vi "TrendsD04.vi"() -> ()   [LabVIEW 2019, in "D04.lvlib"]
uses:
  D04.lvlib
  <vilib>/measure/mamon.llb/Trigger Detection for 1 Channel.vi
  <vilib>/measure/NI_MAPro.lvlib
panel:
  out "No Change":bool
  out "Sudden Change":bool
  out "Decrease":bool
  out "Increase":bool
  out "Previous  ES":dbl
  out "Present  Speed":dbl
  out "Present Error":dbl format="%#.2g"
  out "Previous Error":dbl
  out "Previous  Speed":dbl
  out "Previous PW":dbl caption="Control Information"
  out "Pulse Trends":waveform(i16)[](graph) caption="Waveform Chart - Dark"
  in  "Close":bool
  out "disc name":string="Disc 04 Trends"
  out "dsgs":string="DSGS"
  out "Speed Trend":waveform(dbl)(graph) caption="Waveform Chart - Dark"
  out "Average Trend":waveform(dbl)[](graph) caption="Waveform Chart - Dark"
  out "Live Trend":waveform(dbl)[](graph) caption="Waveform Chart - Dark"
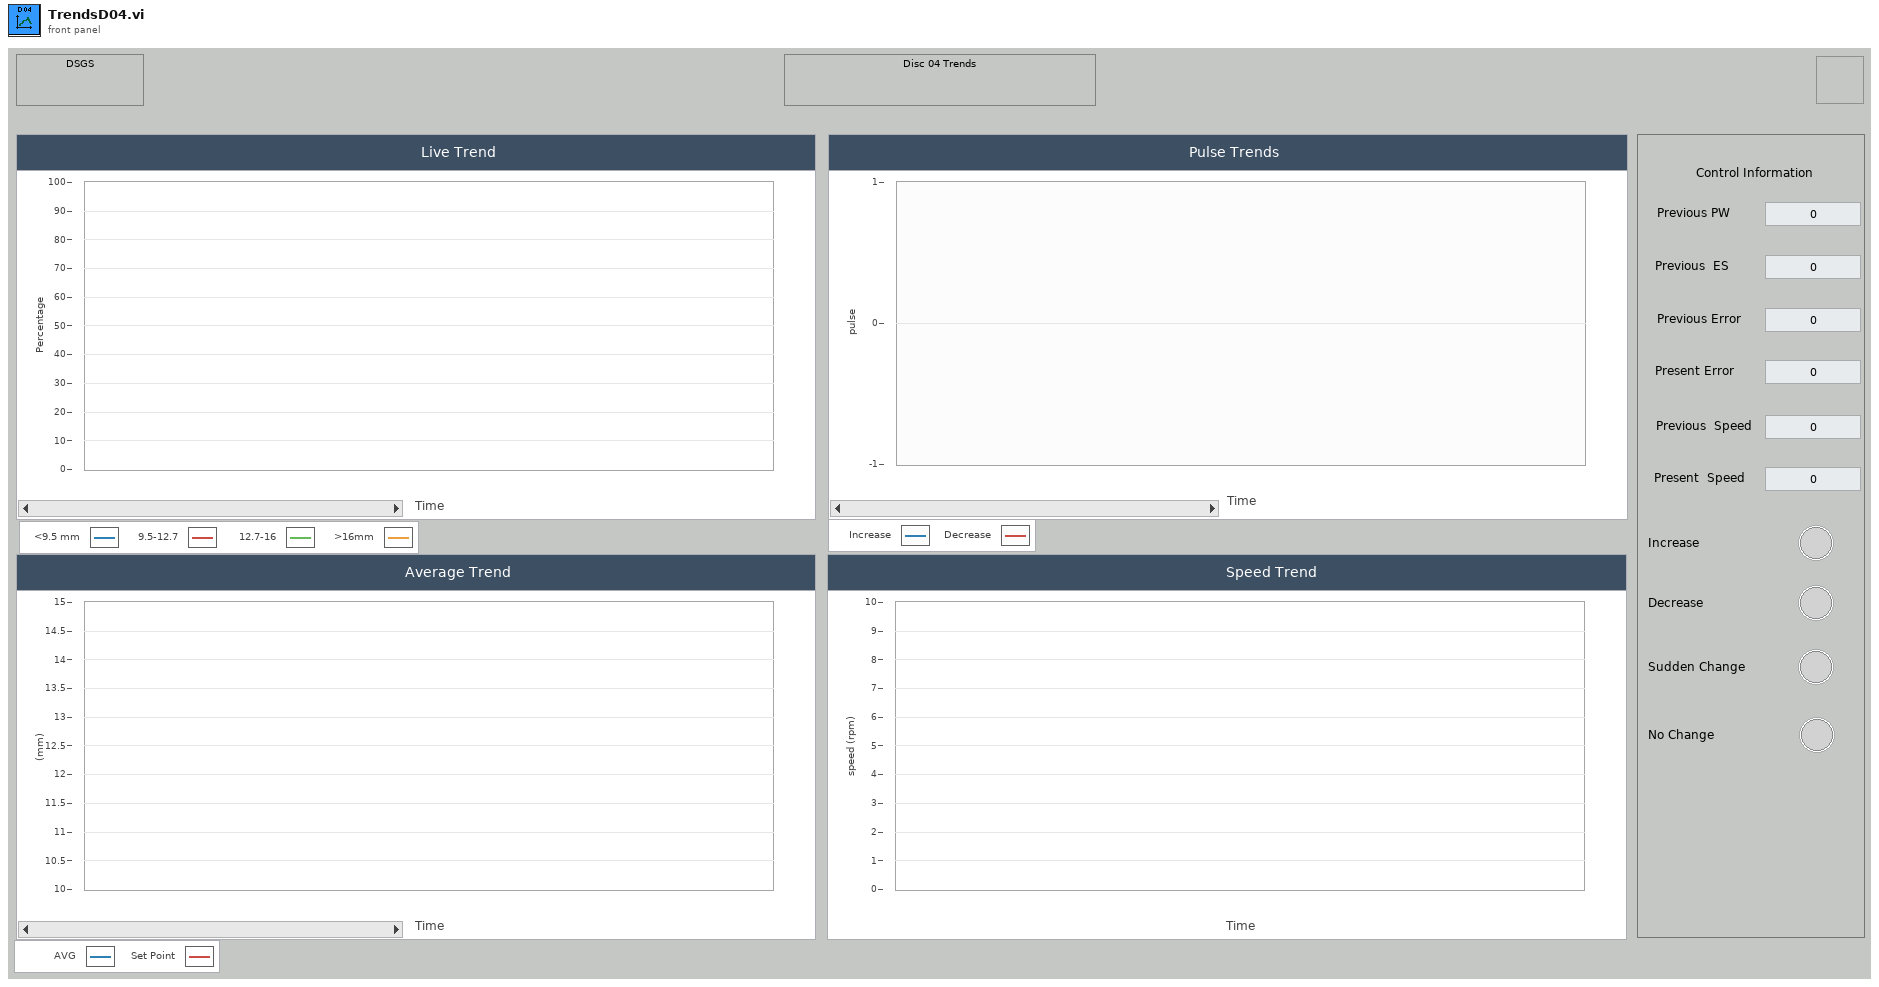
[diagram p1: front panel]
types:
  T1 = cluster{"decrease D04":bool, "increase D04":bool, "no change D04":bool, "sudden change D04":bool, "last error 04":dbl, "previouse speed D04":dbl, "pulse width D04":dbl, "slope D04":dbl}
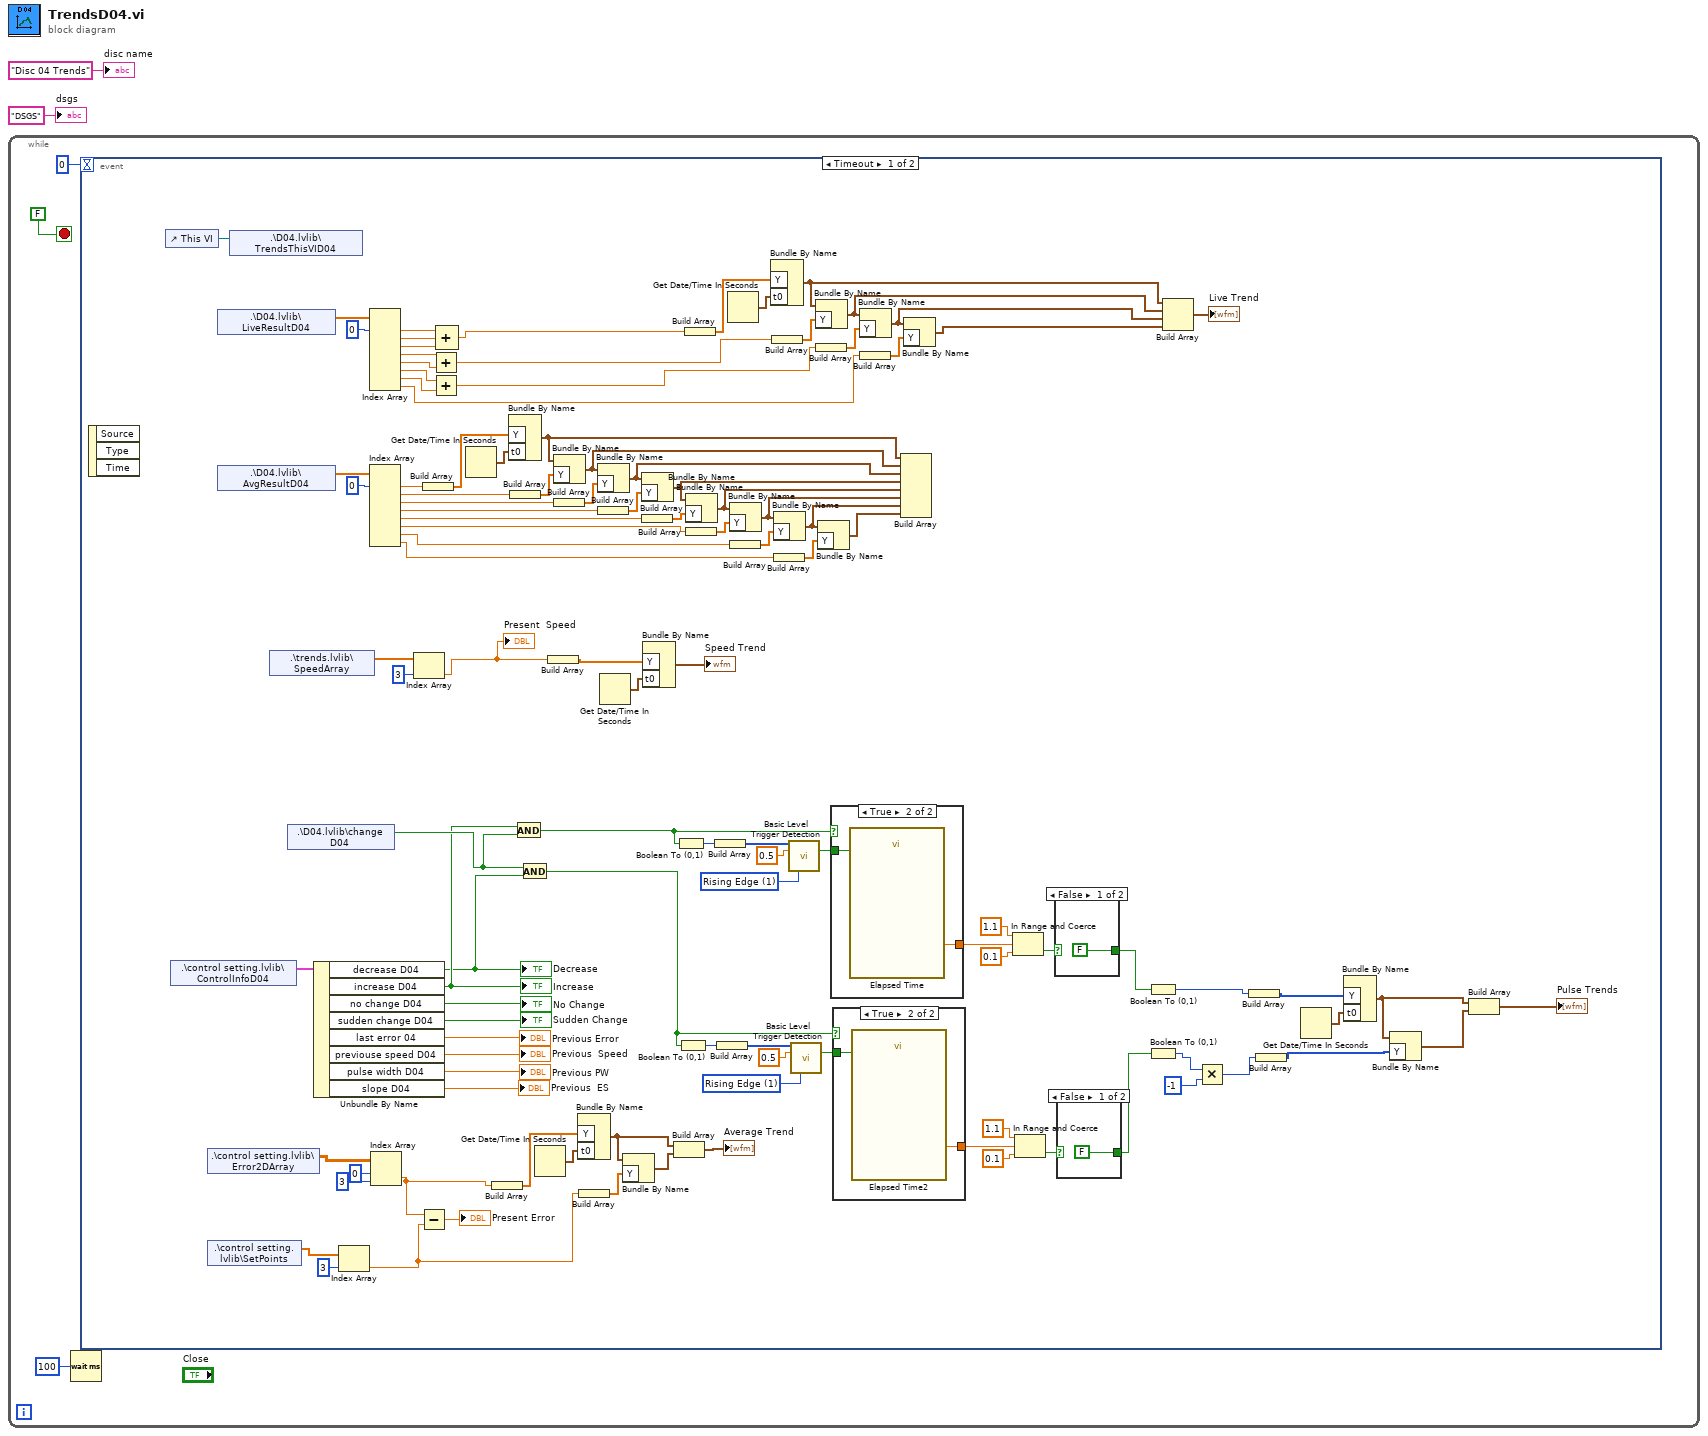
[diagram p0: block diagram]
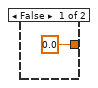
[diagram p3: hidden frame]
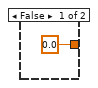
[diagram p5: hidden frame]
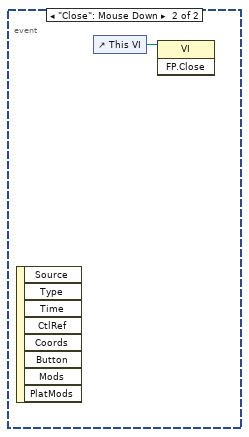
[diagram p6: hidden frame]
diagram:
  n1 = while {
    stop <- FALSE stop-if-true
    n2 = Wait (ms)(milliseconds to wait=u32 100) -> ()  [unwired: 1 out]
    n3 = event shown="[0] Timeout" {
      selector: _ -> [_ _]
      dyn-events: _ -> [_ _]
      timeout: 0 -> [_ _]
      event Timeout {
        w27 = u16 1 items=["Falling Edge", "Rising Edge"] ("trigger slope")
        w38 = u16 1 items=["Falling Edge", "Rising Edge"] ("trigger slope")
        n4 = event-data() -> ()  [unwired: 1 in, 3 out]
        n5 = control-ref of="This VI"() -> (w79:refnum<vi>)
        n6 = shared-variable ".\\control setting.lvlib\\ControlInfoD04"() -> (w63:T1)  [unwired: 1 in, 1 out]
        n7 = shared-variable ".\\control setting.lvlib\\Error2DArray"() -> (w56:dbl[][])  [unwired: 1 in, 1 out]
        n8 = shared-variable ".\\control setting.lvlib\\SetPoints"() -> (w53:dbl[])  [unwired: 1 in, 1 out]
        n9 = shared-variable ".\\D04.lvlib\\LiveResultD04"() -> (w118:dbl[])  [unwired: 1 in, 1 out]
        n10 = shared-variable ".\\D04.lvlib\\AvgResultD04"() -> (w85:dbl[])  [unwired: 1 in, 1 out]
        n11 = shared-variable ".\\D04.lvlib\\TrendsThisVID04"(w79) -> ()  [unwired: 1 in, 1 out]
        n12 = shared-variable ".\\trends.lvlib\\SpeedArray"() -> (w68:dbl[])  [unwired: 1 in, 1 out]
        n13 = shared-variable ".\\D04.lvlib\\change D04"() -> (w49:bool)  [unwired: 1 in, 1 out]
        n14 = Unbundle By Name(w63) -> ("decrease D04"=w47:bool, "increase D04"=w48:bool, "no change D04"=→"No Change":bool, "sudden change D04"=→"Sudden Change":bool, "last error 04"=→"Previous Error":dbl, "previouse speed D04"=→"Previous  Speed":dbl, "pulse width D04"=→"Previous PW":dbl, "slope D04"=→"Previous  ES":dbl)
        "Increase" <- w48
        "Decrease" <- w47
        n15 = Index Array(array=w53, index=3) -> (element=w20:dbl)
        n16 = Index Array(array=w118, index #1=0 ("index")) -> (element #1=w19:dbl, element #2=w18:dbl, element #3=w17:dbl, element #4=w15:dbl, element #5=w14:dbl, element #6=w13:dbl, element #7=w12:dbl, element #8=w9:dbl)  [unwired: 7 in]
        n17 = Index Array(array=w85, index #1=0 ("index")) -> (element #1=w95:dbl, element #2=w96:dbl, element #3=w98:dbl, element #4=w100:dbl, element #5=w101:dbl, element #6=w103:dbl, element #7=w105:dbl, element #8=w83:dbl)  [unwired: 7 in]
        n18 = Index Array(array=w56, index (row)=0, index (col)=3 ("disabled index (col)")) -> (element=w21:dbl)
        n19 = Index Array(array=w68, index=3) -> (element=w50:dbl)
        "Present  Speed" <- w50
        n20 = Subtract(x=w21, y=w20) -> (x-y=→"Present Error":dbl)
        n21 = Build Array(w95) -> (w106:dbl[])
        n22 = Add(x=w15, y=w14) -> (x+y=w11:dbl)
        n23 = Add(x=w13, y=w12) -> (x+y=w10:dbl)
        n24 = Compound Arithmetic op=ADD(w19, w18, w17) -> (w16:dbl)
        n25 = Get Date/Time In Seconds() -> (seconds since 1Jan1904=w88:timestamp)
        n26 = Build Array(w21) -> (w22:dbl[])
        n27 = Bundle By Name("Y"=w106, "t0"=w88) -> (w94:waveform(dbl))  [unwired: 1 in]
        n28 = Build Array(w96) -> (w97:dbl[])
        n29 = And(x=w48, y=w49) -> (x .and. y?=w37:bool)
        n30 = And(x=w49, y=w47) -> (x .and. y?=w26:bool)
        n31 = Get Date/Time In Seconds() -> (seconds since 1Jan1904=w24:timestamp)
        n32 = Build Array(w50) -> (w66:dbl[])
        n33 = Bundle By Name(cluster=w94, "Y"=w97) -> (w93:waveform(dbl))
        n34 = Build Array(w98) -> (w99:dbl[])
        n35 = Bundle By Name("Y"=w22, "t0"=w24) -> (w8:waveform(dbl))  [unwired: 1 in]
        n36 = Build Array(w20) -> (w23:dbl[])
        n37 = Bundle By Name(cluster=w93, "Y"=w99) -> (w92:waveform(dbl))
        n38 = Build Array(w100) -> (w87:dbl[])
        n39 = Get Date/Time In Seconds() -> (seconds since 1Jan1904=w65:timestamp)
        n40 = Bundle By Name(cluster=w8, "Y"=w23) -> (w7:waveform(dbl))
        n41 = Bundle By Name(cluster=w92, "Y"=w87) -> (w91:waveform(dbl))
        n42 = Build Array(w101) -> (w102:dbl[])
        n43 = Bundle By Name("Y"=w66, "t0"=w65) -> (→"Speed Trend":waveform(dbl))  [unwired: 1 in]
        n44 = Build Array(w8, w7) -> (→"Average Trend":waveform(dbl)[])
        n45 = Boolean To (0,1)(Boolean=w37) -> (0, 1=w46:i16)
        n46 = Boolean To (0,1)(Boolean=w26) -> (0, 1=w35:i16)
        n47 = Build Array(w16) -> (w108:dbl[])
        n48 = Bundle By Name(cluster=w91, "Y"=w102) -> (w90:waveform(dbl))
        n49 = Build Array(w103) -> (w104:dbl[])
        n50 = Build Array(w46) -> (w45:i16[])
        n51 = Build Array(w35) -> (w34:i16[])
        n52 = Get Date/Time In Seconds() -> (seconds since 1Jan1904=w115:timestamp)
        n53 = Bundle By Name(cluster=w90, "Y"=w104) -> (w89:waveform(dbl))
        n54 = Build Array(w105) -> (w107:dbl[])
        n55 = Bundle By Name("Y"=w108, "t0"=w115) -> (w111:waveform(dbl))  [unwired: 1 in]
        n56 = Build Array(w11) -> (w110:dbl[])
        n57 = Bundle By Name(cluster=w89, "Y"=w107) -> (w80:waveform(dbl))
        n58 = Build Array(w83) -> (w84:dbl[])
        n59 = call-poly <vilib>:"Basic Level Trigger Detection.vi"("signal in"=w45, "level"=0.5, "trigger slope"=w38) -> ("trigger detected?"=w40:bool)  [unwired: 10 in, 2 out]
        n60 = call-poly <vilib>:"Basic Level Trigger Detection.vi"("signal in"=w34, "level"=0.5, "trigger slope"=w27) -> ("trigger detected?"=w29:bool)  [unwired: 10 in, 2 out]
        n61 = Bundle By Name(cluster=w111, "Y"=w110) -> (w112:waveform(dbl))
        n62 = Build Array(w10) -> (w109:dbl[])
        n63 = Bundle By Name(cluster=w80, "Y"=w84) -> (w82:waveform(dbl))
        n64 = case shown="True" w37 {
          tunnel: [0.0 ("Elapsed Time (s)") w128] -> w43
          tunnel: w40 -> [_ w127]
          frame False {
          }
          frame True {
            n65 = call "Elapsed Time"("Reset"=w127) -> ("Elapsed Time (s)"=w128:dbl)  [unwired: 11 in, 7 out]
          }
        }
        n66 = case shown="True" w26 {
          tunnel: [0.0 ("Elapsed Time (s)") w123] -> w32
          tunnel: w29 -> [_ w122]
          frame False {
          }
          frame True {
            n67 = call "Elapsed Time2"("Reset"=w122) -> ("Elapsed Time (s)"=w123:dbl)  [unwired: 11 in, 7 out]
          }
        }
        n68 = Bundle By Name(cluster=w112, "Y"=w109) -> (w113:waveform(dbl))
        n69 = Build Array(w9) -> (w116:dbl[])
        n70 = Build Array(w94, w93, w92, w91, w90, w89, w80, w82) -> ()  [unwired: 1 out]
        n71 = Bundle By Name(cluster=w113, "Y"=w116) -> (w114:waveform(dbl))
        n72 = In Range and Coerce(upper limit=1.1, x=w43, lower limit=0.1) -> (In Range?=w39:bool)  [unwired: 1 out]
        n73 = In Range and Coerce(upper limit=1.1, x=w32, lower limit=0.1) -> (In Range?=w28:bool)  [unwired: 1 out]
        n74 = case shown="False" w39 {
          selector: w39 -> [_ w125]
          tunnel: [FALSE w125] -> w36
          frame False {
          }
          frame True {
          }
        }
        n75 = case shown="False" w28 {
          selector: w28 -> [_ w120]
          tunnel: [FALSE w120] -> w25
          frame False {
          }
          frame True {
          }
        }
        n76 = Boolean To (0,1)(Boolean=w36) -> (0, 1=w76:i16)
        n77 = Boolean To (0,1)(Boolean=w25) -> (0, 1=w72:i16)
        n78 = Build Array(w111, w112, w113, w114) -> (→"Live Trend":waveform(dbl)[])
        n79 = Multiply(x=w72, y=i16 -1 ("0, 1")) -> (x*y=w70:i16)
        n80 = Build Array(w76) -> (w77:i16[])
        n81 = Build Array(w70) -> (w75:i16[])
        n82 = Get Date/Time In Seconds() -> (seconds since 1Jan1904=w78:timestamp)
        n83 = Bundle By Name("Y"=w77, "t0"=w78) -> (w74:waveform(i16))  [unwired: 1 in]
        n84 = Bundle By Name(cluster=w74, "Y"=w75) -> (w73:waveform(i16))
        n85 = Build Array(w74, w73) -> (→"Pulse Trends":waveform(i16)[])
      }
      event "Close": Mouse Down {
        n86 = event-data() -> ()  [unwired: 1 in, 8 out]
        n87 = control-ref of="This VI"() -> (w129:refnum<vi>)
        n88 = invoke class="VI" method="FP.Close"(reference=w129) -> ()  [unwired: 2 in, 3 out]
      }
    }
  }
  "dsgs" <- "DSGS" ("dsgs")
  "disc name" <- "Disc 04 Trends" ("disc name")
